vi "AIT 1553 - Find Active Busses.vi"(0 "Device Item Ref in":T1 format="%.0x", 11 "error in (no error)":errorcluster) -> (4 "Device Item Ref out":T1 format="%.0x", 6 "Child Refs - 1553 Busses":T1[](array[typedef]) format="%.0x", 15 "error out":errorcluster)   [LabVIEW 2013]
uses:
  <vilib>/NI Veristand/Custom Device API/Custom Device Item Ref.ctl
  <vilib>/NI Veristand/Custom Device Tools/Custom Device Utility Library/RT Debug String Color Spec.ctl
  <vilib>/NI Veristand/Custom Device API/Custom Device API.lvlib
  <vilib>/NI Veristand/Custom Device Tools/Custom Device Utility Library/Custom Device Utility Library.lvlib
panel:
  in  "Bus Page Item Ref":T1 format="%.0x"
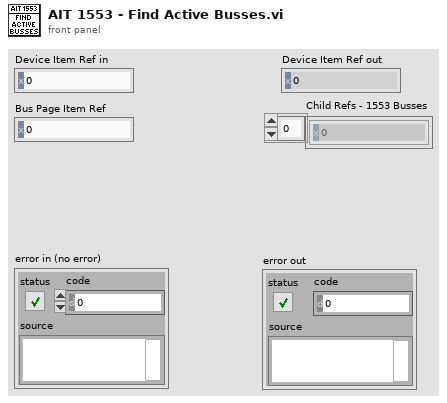
[diagram p1: front panel]
types:
  T1 = typedef "Custom Device API.lvlib/Custom Device Item Ref.ctl" = u64
  T2 = typedef "Custom Device API.lvlib/Custom Device Item Info.ctl" = cluster{"Name":string, "Is Channel":bool, "GUID":string, "Is Waveform":bool}
  T3 = typedef "Custom Device Utility Library.lvlib/RT Debug String Color Spec.ctl" = u16
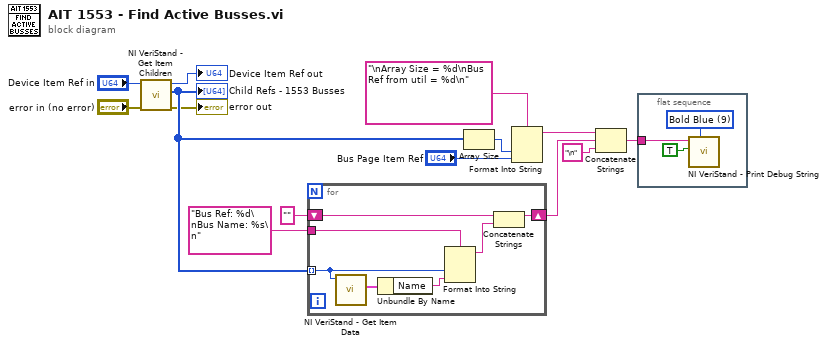
[diagram p0: block diagram]
diagram:
  n1 = call <vilib>:"NI VeriStand - Get Item Children.vi"("error in (no error)"="error in (no error)", "Item Ref in"="Device Item Ref in") -> ("error out"=→"error out":errorcluster, "Child Refs"=w12:T1[], "Item Ref out"=→"Device Item Ref out":T1)  [unwired: 6 in, 1 out]
  "Child Refs - 1553 Busses" <- w12
  n2 = for {
    tunnel: "Bus Ref: %d\nBus Name: %s\n" ("format string") -> [w21]
    tunnel: w12 -> [w18] mode=indexing
    shift-right: [w15] -> w13
    shift-left: "" -> [w20]
    n3 = call <vilib>:"NI VeriStand - Get Item Data.vi"("Item Ref in"=w18) -> ("Item Info"=w17:T2)  [unwired: 1 in, 9 out]
    n4 = Unbundle By Name(w17) -> ("Name"=w16:string)
    n5 = Format Into String(format string=w21, w18, w16) -> (resulting string=w19:string)  [unwired: 2 in, 1 out]
    n6 = Concatenate Strings(w20, w19) -> (w15:string)
  }
  n7 = Array Size(array=w12) -> (size(s)=w11:i32)
  n8 = Format Into String(format string="\nArray Size = %d\nBus Ref from util = %d\n", w11, "Bus Page Item Ref") -> (resulting string=w10:string)  [unwired: 2 in, 1 out]
  n9 = Concatenate Strings(w10, w13, "\n" ("format string")) -> (w9:string)
  n10 = flat-sequence {
    tunnel: w9 -> [w24]
    frame #0 {
      w23 = T3 9 items=["Plain White"=7, "Bold White"=15, "Bold Blue"=9, "Bold Green"=10, "Bold Red"=12] ("Attribute")
      n11 = call <vilib>:"NI VeriStand - Print Debug String.vi"("Attribute"=w23, "Add to log file? (T)"=TRUE, "Message"=w24) -> ()  [unwired: 8 in, 1 out]
    }
  }
